vi "SetPin.vi"(0 "Simulated Device in":refnum<class "Simulated Device.lvclass">, 5 "Port":u8, 7 "Pin":u8, 9 "Value":bool, 11 "error in (no error)":errorcluster) -> (4 "Simulated Device out":refnum<class "Simulated Device.lvclass">, 15 "error out":errorcluster)   [LabVIEW 2020, in "Simulated Device.lvclass"]
doc: "Sends a command to write on a pin of the target device."
uses:
  Simulated Device.lvclass
  Controls/Device Command Code.ctl
  Controls/Device Code.ctl
  <vilib>/Utility/error.llb/Error Cluster From Error Code.vi
  <vilib>/ErrorRing/Error Ring.xnode
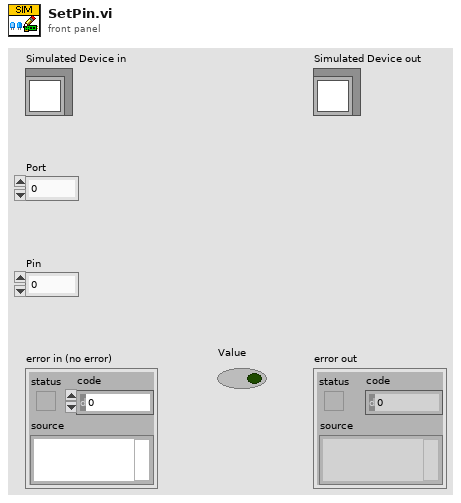
[diagram p1: front panel]
types:
  T1 = typedef "Device Code.ctl" = string
  T2 = typedef "Device Command Code.ctl" = string
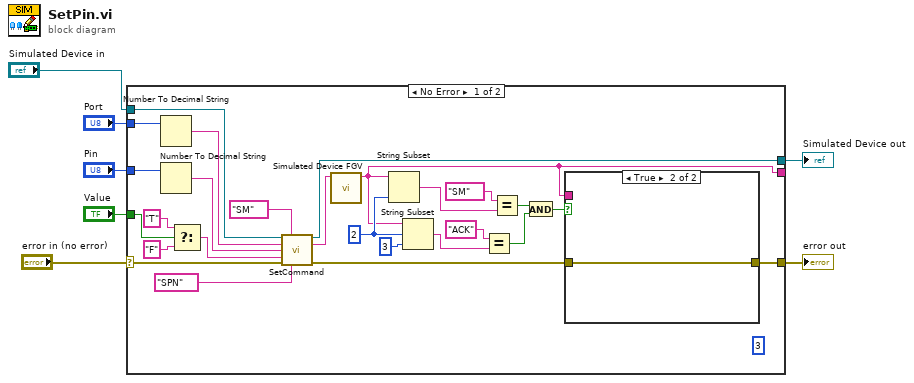
[diagram p0: block diagram]
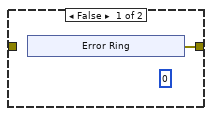
[diagram p2: hidden frame]
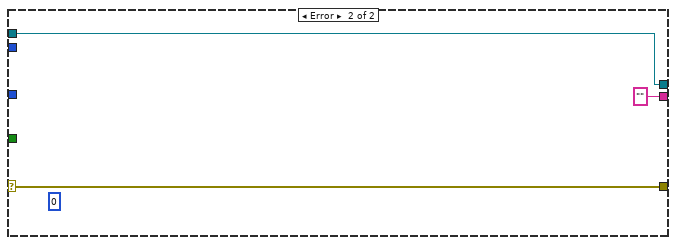
[diagram p3: hidden frame]
diagram:
  n1 = case shown="No Error" "error in (no error)" {
    selector: "error in (no error)" -> [w33 w42]
    tunnel: [w21 w42] -> w1
    tunnel: "Simulated Device in" -> [w31 w43]
    tunnel: [w27 w43] -> w2
    tunnel: "Port" -> [w29 _]
    tunnel: [w8 "" ("read buffer")] -> _
    tunnel: "Pin" -> [w16 _]
    tunnel: "Value" -> [w14 _]
    frame No Error {
      (unwired) 3 ("length (rest)")
      w25 = 2 ("length (rest)")
      n2 = Number To Decimal String(number=w29) -> (decimal integer string=w28:string)  [unwired: 1 in]
      n3 = Number To Decimal String(number=w16) -> (decimal integer string=w15:string)  [unwired: 1 in]
      n4 = Select(t="T", s=w14, f="F") -> (s? t:f=w11:string)
      n5 = call-dynamic "SetCommand.vi"("Simulated Device in"=w31, "Device Code"=T1 "SM", "Parameter 1"=w28, "Parameter 2"=w15, "Parameter 3"=w11, "error in (no error)"=w33, "Command Code"=T2 "SPN") -> ("Simulated Device out"=w27:refnum<class "Simulated Device.lvclass">, "Command"=w9:string, "error out"=w17:errorcluster)  [unwired: 6 in]
      n6 = call "Simulated Device FGV.vi"("Request"=w9) -> ("Response"=w8:string)  [unwired: 10 in]
      n7 = String Subset(string=w8, length (rest)=w25) -> (substring=w19:string)  [unwired: 1 in]
      n8 = String Subset(string=w8, offset (0)=w25, length (rest)=3 ("length (rest)")) -> (substring=w26:string)
      n9 = Equal?(x="ACK", y=w26) -> (x = y?=w23:bool)
      n10 = Equal?(x=T1 "SM" ("Device Code"), y=w19) -> (x = y?=w20:bool)
      n11 = And(x=w20, y=w23) -> (x .and. y?=w22:bool)
      n12 = case shown="True" w22 {
        tunnel: w17 -> [_ w40]
        tunnel: [w34 w40] -> w21
        tunnel: w8 -> [_ _]
        frame False {
          (unwired) u8 0
          n13 = xnode "Error Ring"() -> ("error out"=w34:errorcluster)
        }
        frame True {
        }
      }
    }
    frame Error {
      (unwired) u8 0
    }
  }
  "error out" <- w1
  "Simulated Device out" <- w2
